vi "S Parameter Unit Convert.vi"(9 "Frequency Array":dbl[](array[numeric]), 10 "Format":string, 11 "Waveform IN":dbl[](array[numeric])) -> (2 "Units":string, 3 "Waveform out":dbl[](array[numeric]))   [LabVIEW 2011]
uses:
  www/tests/S Parameter/TypeDefs/SP Format.ctl
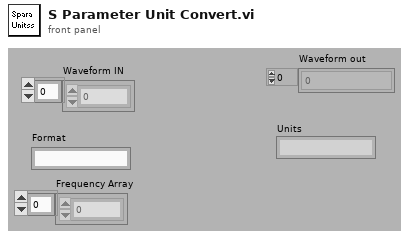
[diagram p1: front panel]
types:
  T1 = typedef "SP Format.ctl" = enum16{"Log Mag", "Lin Mag", "SWR", "Phase", "Expanded Phase", "Delay", "Insertion Loss", "Isolation", "Return Loss"}
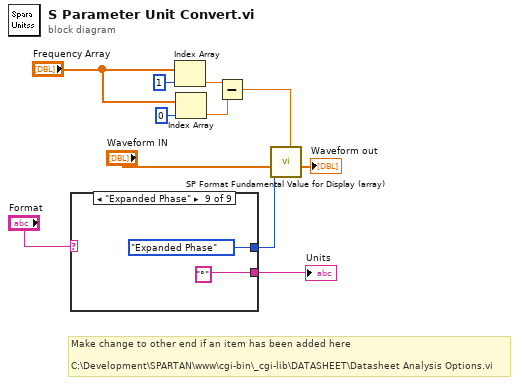
[diagram p0: block diagram]
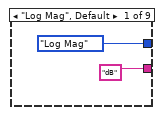
[diagram p2: hidden frame]
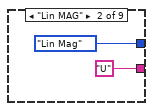
[diagram p3: hidden frame]
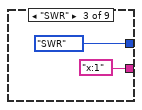
[diagram p4: hidden frame]
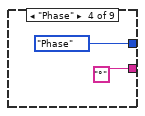
[diagram p5: hidden frame]
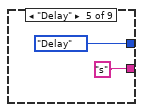
[diagram p6: hidden frame]
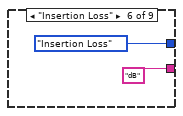
[diagram p7: hidden frame]
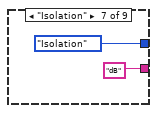
[diagram p8: hidden frame]
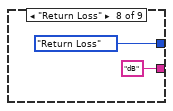
[diagram p9: hidden frame]
diagram:
  # "Make change to other end if an item has been added here\n\nC:\\Development\\SPARTAN\\www\\cgi-bin\\_cgi-lib\\DATASHEET\\Datasheet Analysis Options.vi"
  n1 = case shown="\"Expanded Phase\"" "Format" {
    tunnel: [SP_Format."Log Mag" ("Display Format") SP_Format."Lin Mag" ("Display Format") SP_Format."SWR" ("Display Format") SP_Format."Phase" ("Display Format") SP_Format."Delay" ("Display Format") SP_Format."Insertion Loss" ("Display Format") SP_Format."Isolation" ("Display Format") SP_Format."Return Loss" ("Display Format") SP_Format."Expanded Phase" ("Display Format")] -> w2
    tunnel: ["dB" "U" "x:1" "°" "s" "dB" "dB" "dB" "°"] -> w1
    frame "Log Mag", Default {
    }
    frame "Lin MAG" {
    }
    frame "SWR" {
    }
    frame "Phase" {
    }
    frame "Delay" {
    }
    frame "Insertion Loss" {
    }
    frame "Isolation" {
    }
    frame "Return Loss" {
    }
    frame "Expanded Phase" {
    }
  }
  "Units" <- w1
  n2 = Index Array(array="Frequency Array", index=1) -> (element=w6:dbl)
  n3 = Index Array(array="Frequency Array", index=0) -> (element=w5:dbl)
  n4 = Subtract(x=w6, y=w5) -> (x-y=w4:dbl)
  n5 = call "SP Format Fundamental Value for Display (array).vi"("dF, MHz"=w4, "Display Format"=w2, "Fundamental Values"="Waveform IN") -> ("Formatted Values"=→"Waveform out":dbl[])  [unwired: 1 in, 7 out]
